vi "Schedule Enqueue.vi"(6 "Priority Message? (F)":bool, 7 "StartTime":timestamp, 8 "error in (no error)":errorcluster, 9 "Message Data":variant, 10 "Message":string, 11 "Queue":refnum<queue>) -> (0 "error out":errorcluster, 3 "Scheduled Enqueuer out":refnum<class "Scheduled Enqueue.lvclass">)   [LabVIEW 2020, in "Scheduled Enqueue.lvclass"]
uses:
  Scheduled Enqueue.lvclass
  support/Message Queue/Message Cluster.ctl
  Scheduled Enqueue.lvclass/Scheduled Enqueue.ctl
  Enqueuer.vi
  support/Message Queue/Message Queue.lvlib
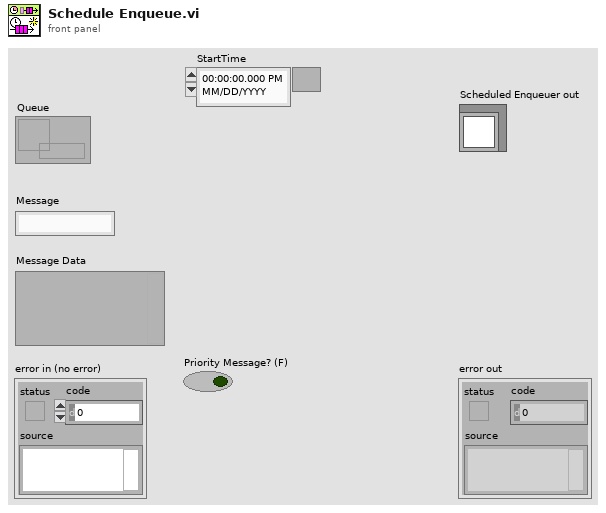
[diagram p1: front panel]
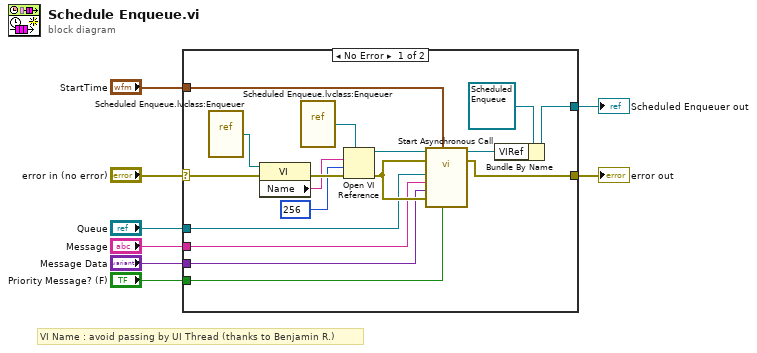
[diagram p0: block diagram]
diagram:
  # "VI Name : avoid passing by UI Thread (thanks to Benjamin R.)"
  n1 = case shown="No Error" "error in (no error)" {
    selector: "error in (no error)" -> [w18 w26]
    tunnel: [w17 w26] -> w7
    tunnel: [w13 _] -> w6
    tunnel: "StartTime" -> [w16 _]
    tunnel: "Queue" -> [w9 _]
    tunnel: "Message" -> [w15 _]
    tunnel: "Message Data" -> [w14 _]
    tunnel: "Priority Message? (F)" -> [w10 _]
    frame No Error {
      n2 = vi-ref "Scheduled Enqueue.lvclass:Enqueuer.vi"() -> (w19:refnum<vi>)
      n3 = property class="VI"(reference=w19, error in=w18) -> (error out=w24:errorcluster, "Name"=w21:string)  [unwired: 1 out]
      n4 = vi-ref "Scheduled Enqueue.lvclass:Enqueuer.vi"() -> (w20:refnum<vi>)
      n5 = Open VI Reference(type specifier VI Refnum (for type only)=w20, vi path=w21, options=256, error in (no error)=w24) -> (vi reference=w23:refnum<vi>, error out=w25:errorcluster)  [unwired: 2 in]
      n6 = call-by-ref "Start Asynchronous Call"(reference=w23, error in=w25, "Priority Message? (F)"=w10, "Start Time"=w16, 8:"error in (no error)"=w25, "Message Data"=w14, "Message"=w15, "Queue"=w9) -> (reference out=w12:refnum<vi>, error out=w17:errorcluster)  [unwired: 5 in, 1 out]
      n7 = Bundle By Name(cluster=refnum<class "Scheduled Enqueue.lvclass"> refnum ("Scheduled Enqueuer in"), "VIRef"=w12) -> (w13:refnum<class "Scheduled Enqueue.lvclass">)
    }
    frame Error {
    }
  }
  "error out" <- w7
  "Scheduled Enqueuer out" <- w6
